vi "SubVI_SingleSymbolRead.vi"(7 "error in (no error)":errorcluster, 9 "SymbolName":string, 10 "Handle":u32) -> (0 "error out":errorcluster, 2 "RData":variant, 3 "Read status?":bool)   [LabVIEW 2022 SP3, in "ADS_Library.lvlib"]
uses:
  ADS_Library.lvlib
  <userlib>/Beckhoff-LabVIEW-Interface/_DependsOn/Base/Read/Read Sync.vi
  <userlib>/Beckhoff-LabVIEW-Interface/_DependsOn/Base/TypeResolver/Get TypeResolver.vi
panel:
  out "RDataArray":variant[](array[variant])
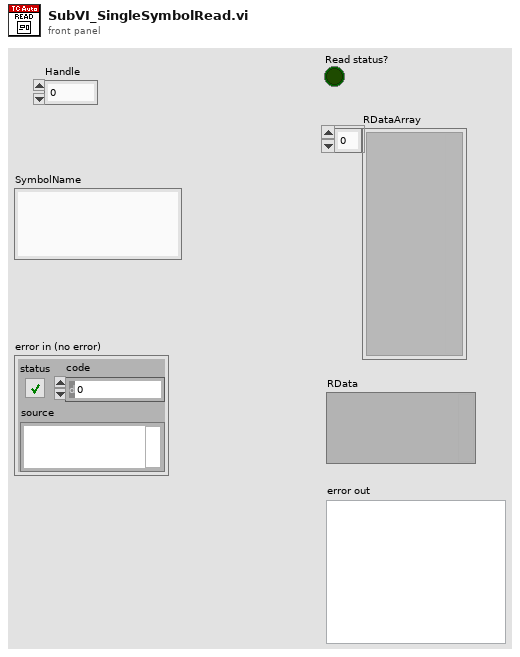
[diagram p1: front panel]
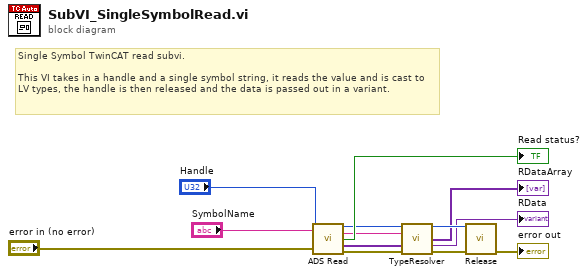
[diagram p0: block diagram]
diagram:
  # "Single Symbol TwinCAT read subvi.\n\nThis VI takes in a handle and a single symbol string, it reads the value and is cast to LV types, the handle is then released and the data is passed out in a variant."
  n1 = call-poly <userlib>:"ADS Read.vi"("Handle"="Handle", "SymbolName"="SymbolName", "error in (no error)"="error in (no error)") -> ("Handle"=w12:u32, "SymbolName"=w11:string, "Read status?"=→"Read status?":bool, "Ads Read Data"=w10:variant[], "error out"=w9:errorcluster)  [unwired: 8 in]
  n2 = call-poly <userlib>:"TypeResolver.vi"("Handle"=w12, "SymbolName"=w11, "ADSRData"=w10, "error in"=w9) -> ("Handle"=w7:u32, "RDataArray"=→"RDataArray":variant[], "RData"=→"RData":variant, "error out"=w8:errorcluster)  [unwired: 8 in]
  n3 = call <userlib>:"Release.vi"("Handle"=w7, "error in (no error)"=w8) -> ("error out"=→"error out":errorcluster)  [unwired: 13 in]
